vi "Khouloud matri (2).vi"() -> ()   [LabVIEW 2015]
panel:
  in  "?":bool
  in  "pump speed":dbl
  out "LLS":bool
  out "HLS":bool
  in  "?":bool
  in  "?":bool
  in  "?":bool
  out "Alarme":bool
  out "Etat":string
  out "Tank":dbl(slide) scale=0.0..10.0
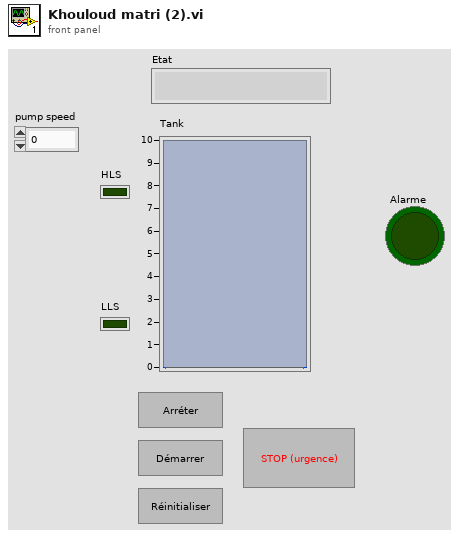
[diagram p1: front panel]
types:
  T1 = enum16{"Arrêt", "Fonctionnement normal", "Alarme"}
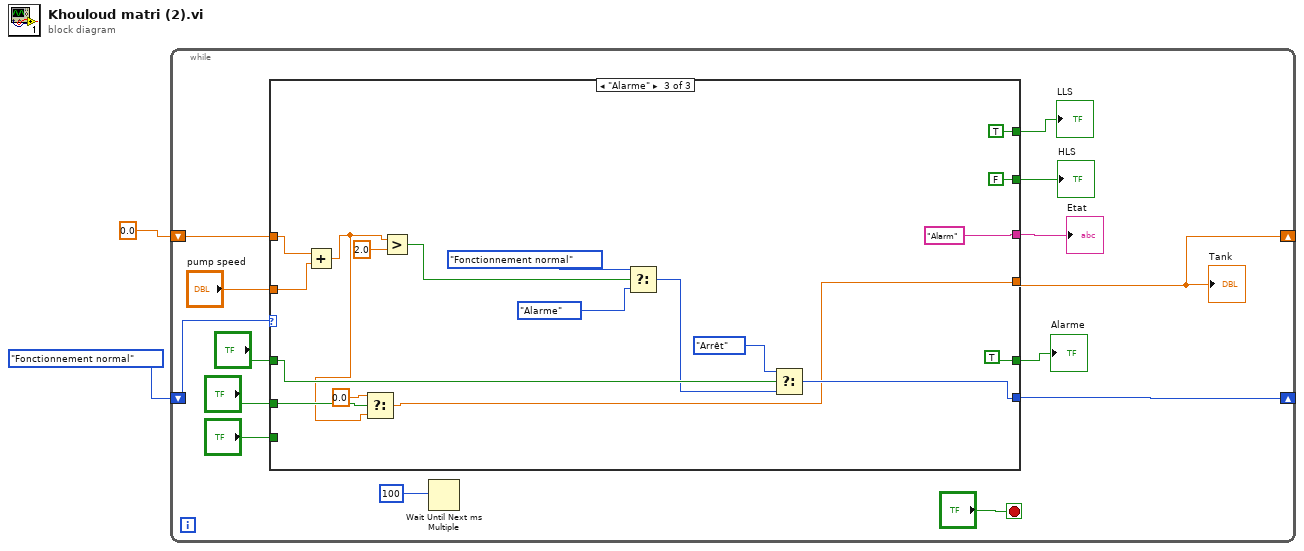
[diagram p0: block diagram]
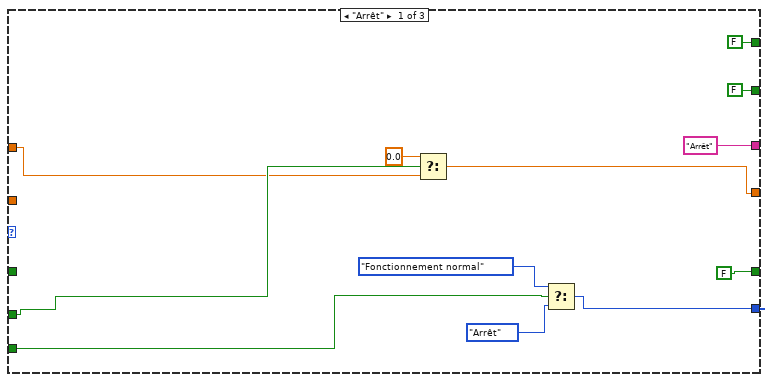
[diagram p2: hidden frame]
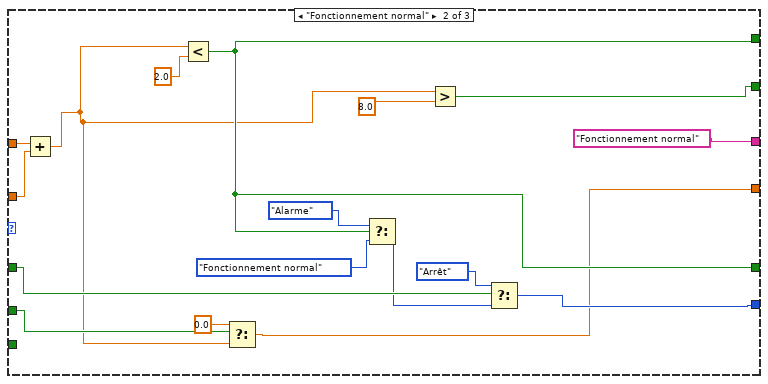
[diagram p3: hidden frame]
diagram:
  n1 = while {
    shift-right: [w15] -> _
    shift-left: T1."Fonctionnement normal" -> [w16]
    shift-right: [w6] -> _
    shift-left: 0.0 ("Capteur") -> [w5]
    stop <- "?" stop-if-true
    n2 = case shown="\"Alarme\"" w16 {
      tunnel: [w26 w40 w57] -> w15
      tunnel: ["Arrêt" "Fonctionnement normal" "Alarm"] -> w14
      tunnel: [w20 w32 w49] -> w6
      tunnel: "?" -> [_ w39 w59]
      tunnel: [FALSE w35 TRUE] -> w11
      tunnel: "?" -> [w21 w34 w50]
      tunnel: [FALSE w36 FALSE] -> w8
      tunnel: [FALSE w35 TRUE] -> w7
      tunnel: w5 -> [w18 w30 w48]
      tunnel: "pump speed" -> [_ w29 w47]
      tunnel: "?" -> [w17 _ _]
      frame "Arrêt" {
        n3 = Select(t=0.0, s=w21, f=w18) -> (s? t:f=w20:dbl)
        n4 = Select(t=T1."Fonctionnement normal", s=w17, f=T1."Arrêt") -> (s? t:f=w26:T1)
      }
      frame "Fonctionnement normal" {
        n5 = Add(x=w30, y=w29) -> (x+y=w31:dbl)
        n6 = Less?(x=w31, y=2.0) -> (x < y?=w35:bool)
        n7 = Select(t=0.0, s=w34, f=w31) -> (s? t:f=w32:dbl)
        n8 = Select(t=T1."Alarme", s=w35, f=T1."Fonctionnement normal") -> (s? t:f=w38:T1)
        n9 = Greater?(x=w31, y=8.0) -> (0:w36:bool)
        n10 = Select(t=T1."Arrêt", s=w39, f=w38) -> (s? t:f=w40:T1)
      }
      frame "Alarme" {
        n11 = Add(x=w48, y=w47) -> (x+y=w46:dbl)
        n12 = Select(t=0.0, s=w50, f=w46) -> (s? t:f=w49:dbl)
        n13 = Greater?(x=w46, y=2.0) -> (0:w55:bool)
        n14 = Select(t=T1."Fonctionnement normal", s=w55, f=T1."Alarme") -> (s? t:f=w58:T1)
        n15 = Select(t=T1."Arrêt", s=w59, f=w58) -> (s? t:f=w57:T1)
      }
    }
    "Etat" <- w14
    "Tank" <- w6
    "Alarme" <- w11
    "HLS" <- w8
    "LLS" <- w7
    n16 = Wait Until Next ms Multiple(millisecond multiple=u32 100 ("milliseconds to wait")) -> ()  [unwired: 1 out]
  }
